vi "testCalcUkInComcam.vi"(8 "error in (no error)":errorcluster) -> (0 "error out":errorcluster)   [LabVIEW 2016]
doc: "Test to calculate uk for ComCam 9 wavefront front sensors (WFSs."
uses:
  ZTAAC/ZTAAC.lvclass
  StrictDef/FilterType.ctl
  StrictDef/InstName.ctl
  <vilib>/Analysis/BLAS.llb/dasum - Absolute Values Sum (DBL).vi
  <vilib>/addons/_JKI Toolkits/Caraya/classes/Test/Test.lvclass
  <vilib>/Analysis/NI_AALBLAS.lvlib
  <vilib>/addons/_JKI Toolkits/Caraya/classes/Assert/Assert.lvclass
  MatOper/MatOper.lvclass
  OfcFunc.lvlib
panel:
  in  "ZTAAC.lvclass":refnum<class "ZTAAC.lvclass">
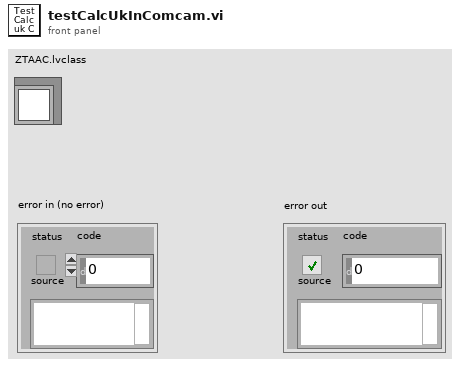
[diagram p1: front panel]
types:
  T1 = typedef "OfcFunc.lvlib/InstName.ctl" = enum16{"lsst", "comcam"}
  T2 = typedef "OfcFunc.lvlib/FilterType.ctl" = enum16{"ref", "u", "g", "r", "i", "z", "y"}
  T3 = cluster{"Config Dir":path, "Inst Name":T1, "OptStateEsti Config File Name":string, "Mapping File Name":string, "Wavelength Table":string, "Intrinc Zk File Name":string, "y2 Corection File Name":string, "Index DOF File Name":string, "OptCtrl Config File Name":string, "State 0 File Name":string, "Weighting File Name":string, "PSSN Alpha File Name":string, "Authority Files":cluster{"Rigid Body Stroke File":string, "M1M3 Subsystem":cluster{"Mirror":string, "Actuatro Force File":string}, "M2 Subsystem":cluster{"Mirror":string, "Actuatro Force File":string}, "Num of Bending Mode":i32}, "Sensor Id to Name File Name":string, "Truncation Threshold":dbl, "Default Gain":dbl, "FWHM Threshold (arcsec)":dbl}
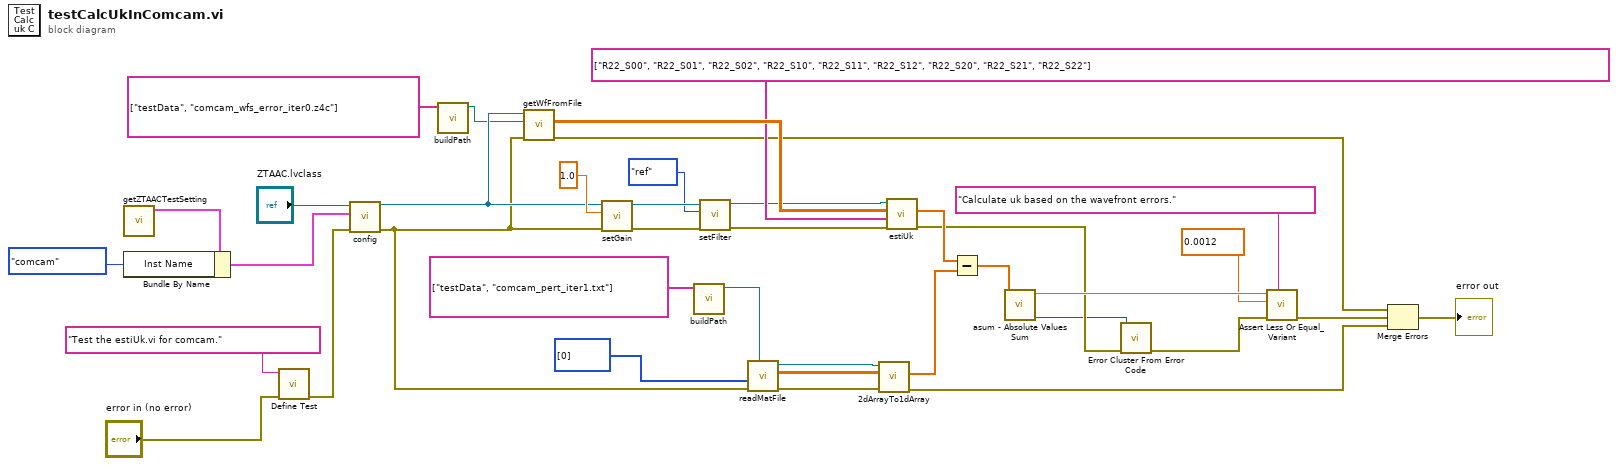
[diagram p0: block diagram]
diagram:
  n1 = call "getZTAACTestSetting.vi"() -> ("Test Setting"=w7:T3)  [unwired: 11 in]
  n2 = Bundle By Name(cluster=w7, "Inst Name"=InstName."comcam") -> (w5:T3)
  n3 = call <vilib>:"Define Test.vi"("error in (no error)"="error in (no error)", "Label (VI Title)"="Test the estiUk.vi for comcam.") -> ("error out"=w31:errorcluster)  [unwired: 9 in]
  n4 = call "config.vi"("error in (no error)"=w31, "ZTAAC Configuration"=w5, "ZTAAC in"="ZTAAC.lvclass") -> ("error out"=w29:errorcluster, "ZTAAC out"=w36:refnum<class "ZTAAC.lvclass">)  [unwired: 7 in]
  n5 = call "buildPath.vi"("Path Name List"=string[] ["testData", "comcam_wfs_error_iter0.z4c"]) -> ("New Path"=w3:path)  [unwired: 10 in]
  n6 = call "getWfFromFile.vi"("error in (no error)"=w29, "Wfs Err Data"=w3, "ZTAAC in"=w36) -> ("error out"=w28:errorcluster, "Wavefront Error"=w35:dbl[][])  [unwired: 6 in, 1 out]
  n7 = call "setGain.vi"("error in (no error)"=w29, "Gain"=1.0, "ZTAAC in"=w36) -> ("error out"=w11:errorcluster, "ZTAAC out"=w12:refnum<class "ZTAAC.lvclass">)  [unwired: 7 in]
  n8 = call "buildPath.vi"("Path Name List"=string[] ["testData", "comcam_pert_iter1.txt"]) -> ("New Path"=w1:path)  [unwired: 10 in]
  n9 = call "setFilter.vi"("error in (no error)"=w11, "Filter Type"=FilterType."ref", "ZTAAC in"=w12) -> ("error out"=w10:errorcluster, "ZTAAC out"=w9:refnum<class "ZTAAC.lvclass">)  [unwired: 7 in]
  n10 = call "readMatFile.vi"("Path"=w1, "error in (no error)"=w29, "Skip Col Idx"=i32[] [0] ("Skip Row Idx")) -> ("error out"=w14:errorcluster, "Matrix"=w33:dbl[][], "MatOper out"=w15:refnum<class "MatOper.lvclass">)  [unwired: 6 in]
  n11 = call "2dArrayTo1dArray.vi"("error in (no error)"=w14, "2D Array"=w33, "MatOper in"=w15) -> ("error out"=w13:errorcluster, "1D Array"=w25:dbl[])  [unwired: 6 in, 1 out]
  n12 = call "estiUk.vi"("error in (no error)"=w10, "Sensor Name"=string[] ["R22_S00", "R22_S01", "R22_S02", "R22_S10", "R22_S11", "R22_S12", "R22_S20", "R22_S21", "R22_S22"], "Wavefront Error"=w35, "ZTAAC in"=w9) -> ("error out"=w21:errorcluster, "uk Array"=w26:dbl[])  [unwired: 5 in, 1 out]
  n13 = Subtract(x=w26, y=w25) -> (x-y=w24:dbl[])
  n14 = call-poly <vilib>:"asum - Absolute Values Sum.vi"("x"=w24) -> ("error"=w20:i32, "dasum"=w23:dbl)  [unwired: 9 in]
  n15 = call <vilib>:"Error Cluster From Error Code.vi"("error in (no error)"=w21, "error code (0)"=w20) -> ("error out"=w19:errorcluster)  [unwired: 7 in]
  n16 = call <vilib>:"Assert Less Or Equal_Variant.vi"("Label"="Calculate uk based on the wavefront errors.", "error in (no error)"=w19, "Y"=0.0012, "X"=w23) -> ("error out"=w18:errorcluster)  [unwired: 7 in]
  n17 = Merge Errors(w28, w18, w13) -> (→"error out":errorcluster)
